vi "PostPersonnel.vi"(7 "LabVIEW Web Service Request":refnum<class "Web Request.lvclass">, 9 "Data":string, 10 "Command":string, 11 "UID":string) -> (2 "Response":string)   [LabVIEW 2015]
uses:
  <vilib>/wsapi/Web Request.lvclass
  TypeDef/PersonnelActions.ctl
  TypeDef/RoomsActionEnum.ctl
panel:
  out "output array":string[](array[string])
  in  "s":bool
  out "current time":timestamp
  out "postdata":string
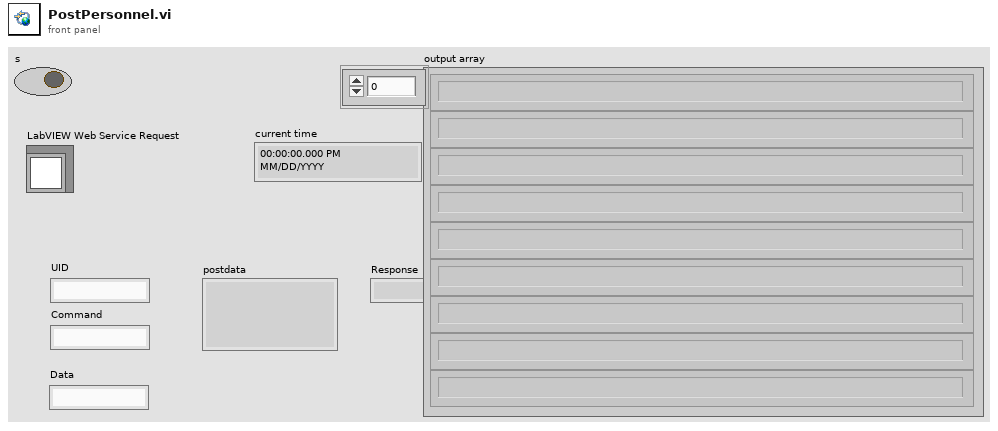
[diagram p1: front panel]
types:
  T1 = typedef "PersonnelActions.ctl" = enum16{"Init", "Read Personnel", "Add Personnel", "Remove Personnel", "Read Name", "Write Name", "Read Role", "Write Role", "Read Requests", "Add Requests", "Remove Requests", "Read PUIDs"}
  T2 = typedef "RoomsActionEnum.ctl" = enum16{"Init", "Add Room", "Remove Room", "Read Room", "Read Flag", "Read Flag State", "Write Flag State", "Read Flag Color", "Write Flag Color", "Read Bed Vacant", "Write Bed Vacant", "Read Personnel", "Add Personnel", "Remove Personnel", "Read Requests", "Add Request", "Remove Request", "Read Beacon ID", "Write Beacon ID", "Write Bed URL", "Read Bed URL", "Read Rooms Numbers", "Write Flag"}
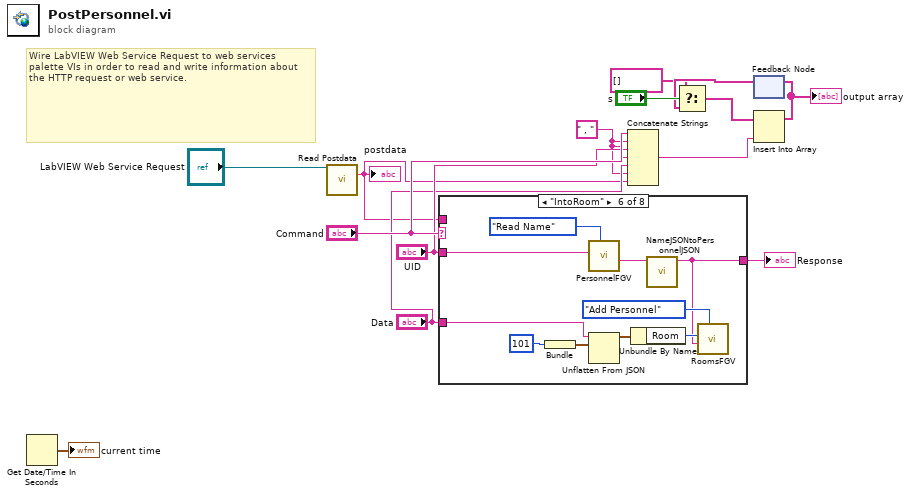
[diagram p0: block diagram]
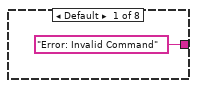
[diagram p2: hidden frame]
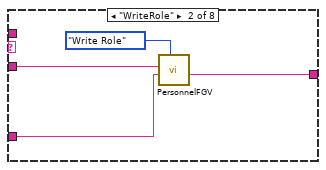
[diagram p3: hidden frame]
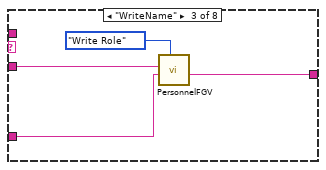
[diagram p4: hidden frame]
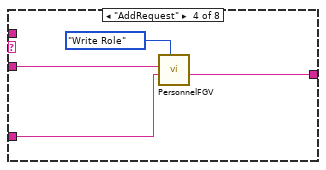
[diagram p5: hidden frame]
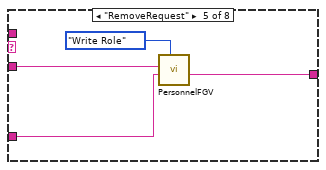
[diagram p6: hidden frame]
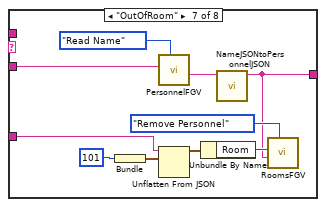
[diagram p7: hidden frame]
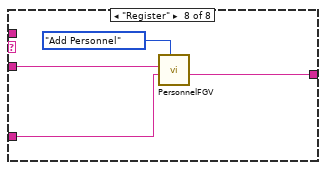
[diagram p8: hidden frame]
diagram:
  w1 = " , " ("string")
  # "Wire LabVIEW Web Service Request to web services palette VIs in order to read and write information about the HTTP request or web service."
  n1 = Get Date/Time In Seconds() -> (seconds since 1Jan1904=→"current time":timestamp)
  n2 = call <vilib>:"Read Postdata.vi"("LabVIEW Web Service Request"="LabVIEW Web Service Request") -> ("postdata"=w8:string)  [unwired: 12 in, 2 out]
  "postdata" <- w8
  n3 = case shown="\"IntoRoom\"" "Command" {
    tunnel: w8 -> [_ _ _ _ _ _ _ _]
    tunnel: "UID" -> [_ w18 w22 w26 w30 w40 w50 w54]
    tunnel: "Data" -> [_ w17 w21 w25 w29 w36 w46 w53]
    tunnel: ["Error: Invalid Command" ("Data Out") w16 w20 w24 w28 w32 w42 w52] -> w13
    frame Default {
    }
    frame "WriteRole" {
      n4 = call "PersonnelFGV.vi"("Actions"=PersonnelActions."Write Role", "Data In"=w17, "PUID"=w18) -> ("Data Out"=w16:string)  [unwired: 7 in, 1 out]
    }
    frame "WriteName" {
      n5 = call "PersonnelFGV.vi"("Actions"=PersonnelActions."Write Role", "Data In"=w21, "PUID"=w22) -> ("Data Out"=w20:string)  [unwired: 7 in, 1 out]
    }
    frame "AddRequest" {
      n6 = call "PersonnelFGV.vi"("Actions"=PersonnelActions."Write Role", "Data In"=w25, "PUID"=w26) -> ("Data Out"=w24:string)  [unwired: 7 in, 1 out]
    }
    frame "RemoveRequest" {
      n7 = call "PersonnelFGV.vi"("Actions"=PersonnelActions."Write Role", "Data In"=w29, "PUID"=w30) -> ("Data Out"=w28:string)  [unwired: 7 in, 1 out]
    }
    frame "IntoRoom" {
      n8 = Bundle("Room"=101) -> (w37:cluster{"Room":i32})  [unwired: 1 in]
      n9 = call "PersonnelFGV.vi"("Actions"=PersonnelActions."Read Name", "PUID"=w40) -> ("Data Out"=w33:string)  [unwired: 8 in, 1 out]
      n10 = Unflatten From JSON(JSON string=w36, type and defaults=w37) -> (value=w35:cluster{"Room":i32})  [unwired: 5 in, 1 out]
      n11 = Unbundle By Name(w35) -> ("Room"=w34:i32)
      n12 = call "NameJSONtoPersonnelJSON.vi"("Name JSON"=w33) -> ("Personnel JSON"=w32:string)  [unwired: 10 in]
      n13 = call "RoomsFGV.vi"("Actions"=RoomsActionEnum."Add Personnel", "Data In"=w32, "Room"=w34) -> ()  [unwired: 7 in, 2 out]
    }
    frame "OutOfRoom" {
      n14 = Bundle("Room"=101) -> (w47:cluster{"Room":i32})  [unwired: 1 in]
      n15 = call "PersonnelFGV.vi"("Actions"=PersonnelActions."Read Name", "PUID"=w50) -> ("Data Out"=w43:string)  [unwired: 8 in, 1 out]
      n16 = Unflatten From JSON(JSON string=w46, type and defaults=w47) -> (value=w45:cluster{"Room":i32})  [unwired: 5 in, 1 out]
      n17 = Unbundle By Name(w45) -> ("Room"=w44:i32)
      n18 = call "NameJSONtoPersonnelJSON.vi"("Name JSON"=w43) -> ("Personnel JSON"=w42:string)  [unwired: 10 in]
      n19 = call "RoomsFGV.vi"("Actions"=RoomsActionEnum."Remove Personnel", "Data In"=w42, "Room"=w44) -> ()  [unwired: 7 in, 2 out]
    }
    frame "Register" {
      n20 = call "PersonnelFGV.vi"("Actions"=PersonnelActions."Add Personnel", "Data In"=w53, "PUID"=w54) -> ("Data Out"=w52:string)  [unwired: 7 in, 1 out]
    }
  }
  "Response" <- w13
  n21 = Concatenate Strings("Command", w1, "UID", w1, "Data", w1, w8) -> (w7:string)
  n22 = feedback #1() -> (w4:string[])  [unwired: 1 in]
  n23 = Select(t=string[] [], s="s", f=w4) -> (s? t:f=w2:string[])
  n24 = Insert Into Array(array=w2, new element=w7) -> (w6:string[])  [unwired: 1 in]
  "output array" <- w6
  n25 = feedback-in #1(w6) -> ()
